vi "S2C_SetDataCmdr.vi"(8 "Error In":errorcluster, 11 "MenuRef":refnum<k9>) -> (0 "Error Out":errorcluster)   [LabVIEW 2015]
doc: "Toggles the \"Local File\" runtime menu item."
uses:
  LVIS/Sub VIs/Globals/LVIS_DcGlobals.vi
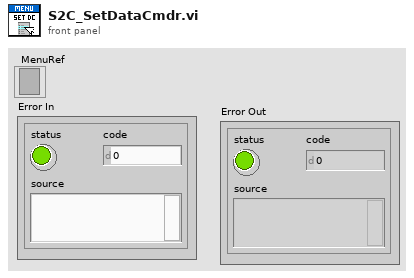
[diagram p1: front panel]
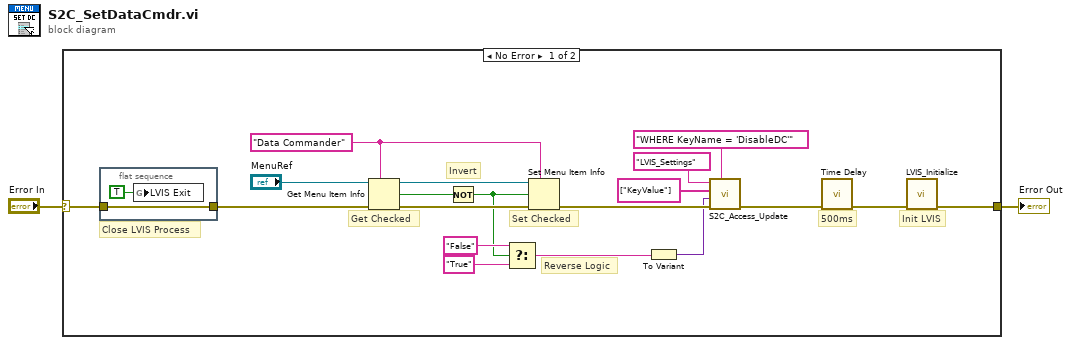
[diagram p0: block diagram]
diagram:
  n1 = case shown="No Error" "Error In" {
    selector: "Error In" -> [w13 w24]
    tunnel: [w11 w24] -> w1
    frame No Error {
      w20 = "Data Commander" ("item tag")
      # "500ms"
      # "Reverse Logic"
      # "Init LVIS"
      # "Close LVIS Process"
      # "Invert"
      # "Set Checked"
      # "Get Checked"
      n2 = flat-sequence {
        tunnel: w13 -> [w22]
        tunnel: [w22] -> w12
        frame #0 {
          n3 = global write "LVIS_DcGlobals.vi" "LVIS Exit"(TRUE ("LVIS Exit")) -> ()
        }
      }
      n4 = Get Menu Item Info(7:w20, 8:w12, 11:"MenuRef") -> (0:w19:errorcluster, 3:w18:refnum<k9>, 4:w17:bool)  [unwired: 4 out]
      n5 = Not(x=w17) -> (.not. x?=w14:bool)
      n6 = Select(t="False", s=w14, f="True") -> (s? t:f=w7:string)
      n7 = Set Menu Item Info(6:w14, 7:w20, 8:w19, 11:w18) -> (0:w9:errorcluster)  [unwired: 3 in, 1 out]
      n8 = To Variant(anything=w7) -> (Variant=w6:variant)
      n9 = call "S2C_Access_Update.vi"("Condition"="WHERE KeyName = 'DisableDC'", "Error In"=w9, "Data"=w6, "Columns"=string[] ["KeyValue"], "Table"="LVIS_Settings") -> ("Error Out"=w5:errorcluster)  [unwired: 6 in]
      n10 = call "Time Delay"("error in (no error)"=w5) -> ("error out"=w10:errorcluster)  [unwired: 10 in]
      n11 = call "LVIS_Initialize.vi"("Error In"=w10) -> ("Error Out"=w11:errorcluster)  [unwired: 9 in, 1 out]
    }
    frame Error {
    }
  }
  "Error Out" <- w1
